vi "Send Packets.vi"(0 "WS Test Server Subscriber in":refnum<class "WS Server Subscriber.lvclass">, 5 "Data To Send":string, 7 "Number of Packets":i32=1, 9 "Send Period (ms)":i32=1000, 11 "error in (no error)":errorcluster) -> (4 "WS Test Server Subscriber out":refnum<class "WS Server Subscriber.lvclass">, 15 "error out":errorcluster)   [LabVIEW 2021, in "Echo Broadcast With Server Manager.lvlib" / "WS Server Subscriber.lvclass"]
uses:
  WS Server Subscriber.lvclass
  C:/Program Files/National Instruments/LabVIEW 2021/vi.lib/ActorFramework/Actor/Actor.lvclass
  Sender Loop/Sender Loop.lvclass
  WS Server Subscriber.lvclass/WS Server Subscriber.ctl
  Sender Loop/Sender Loop.lvclass/Sender Loop.ctl
  Sender Loop/properties/Write Data To Send.vi
  Sender Loop/properties/Write Number of Packets.vi
  Sender Loop/properties/Write Send Period (ms).vi
  Sender Loop/properties/Write WebSocket Service Enqueuer.vi
  <vilib>/ActorFramework/Actor/Actor.lvclass
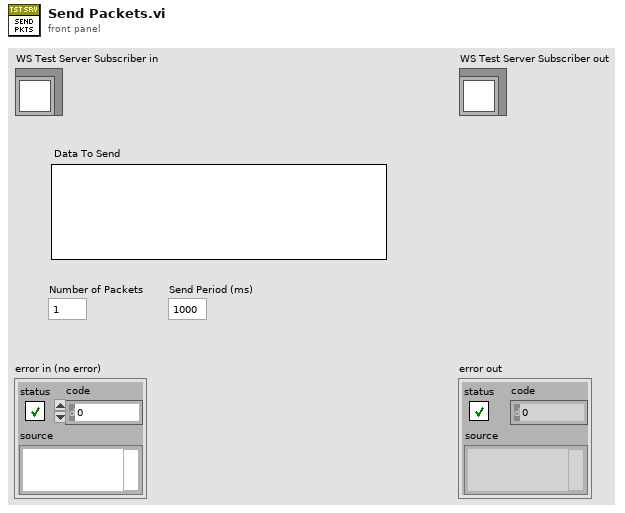
[diagram p1: front panel]
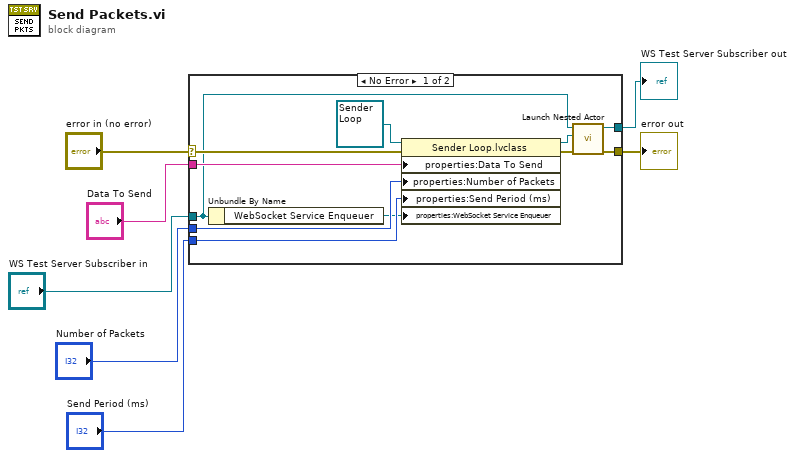
[diagram p0: block diagram]
diagram:
  n1 = case shown="No Error" "error in (no error)" {
    selector: "error in (no error)" -> [w14 w20]
    tunnel: [w13 w20] -> w6
    tunnel: [w15 w19] -> w4
    tunnel: "WS Test Server Subscriber in" -> [w9 w19]
    tunnel: "Data To Send" -> [w12 _]
    tunnel: "Number of Packets" -> [w11 _]
    tunnel: "Send Period (ms)" -> [w10 _]
    frame No Error {
      n2 = Unbundle By Name(w9) -> ("WebSocket Service Enqueuer"=w8:refnum<class "Message Enqueuer.lvclass">)
      n3 = property class="Sender Loop.lvclass"(reference=refnum<class "Sender Loop.lvclass"> refnum ("Echo Broadcast Test With Server Manager.lvlib:Sender Loop.lvclass"), error in=w14, "properties:Data To Send"=w12, "properties:Number of Packets"=w11, "properties:Send Period (ms)"=w10, "properties:WebSocket Service Enqueuer"=w8) -> (reference out=w16:refnum<class "Sender Loop.lvclass">, error out=w17:errorcluster)
      n4 = call <vilib>:"Launch Nested Actor.vi"("error in (no error)"=w17, "Nested Actor"=w16, "Caller Actor in"=w9) -> ("error out"=w13:errorcluster, "Caller Actor out"=w15:refnum<class "WS Server Subscriber.lvclass">)  [unwired: 6 in, 1 out]
    }
    frame Error {
    }
  }
  "error out" <- w6
  "WS Test Server Subscriber out" <- w4
